vi "SCA state Transition Timeout Check.vi"(6 "Start Time":u32, 9 "Timeout limit":u32, 10 "Current State In":T1, 11 "Modified Array of states in":T1[](array[typedef])) -> (0 "Status Message":string, 1 "millisecond timer value out":u32, 2 "Next State":T1, 3 "Modified Array of states out":T1[](array[typedef]))   [LabVIEW 2016]
doc: "Tranision Timeout Check takes the current state, modified array of states, timeout limit, and start time to: \n\n(1) determine if process has timed out\n(2) what state to progress to next, and \n(3) what the current status message should be."
uses:
  controls/SCA states.ctl
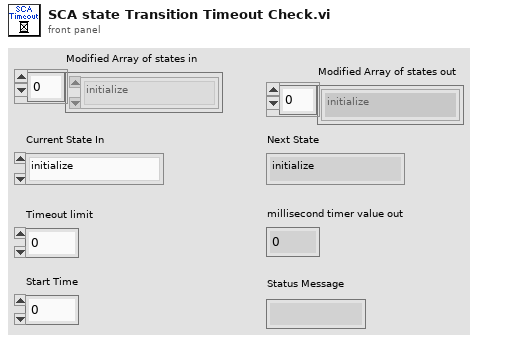
[diagram p1: front panel]
types:
  T1 = typedef "SCA states.ctl" = enum16{"initialize", "wait", "change sample start", "change sample", "check position", "rotate wheel", "sample change complete", "sample rod up", "sample rod down", "retract rod in", "retract rod out", "insert rod in", "insert rod out", "wheel GV open", "wheel GV close", "vent source", "pump source", "shutdown"}
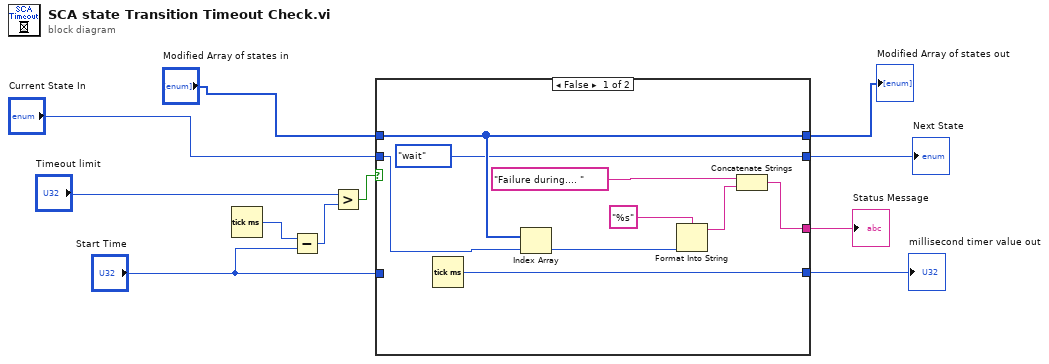
[diagram p0: block diagram]
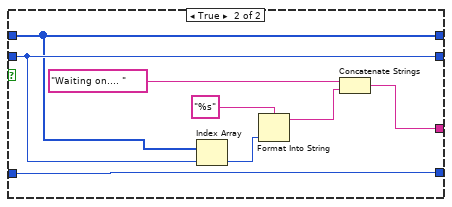
[diagram p2: hidden frame]
diagram:
  n1 = Tick Count (ms)() -> (millisecond timer value=w6:u32)
  n2 = Subtract(x=w6, y="Start Time") -> (x-y=w7:u32)
  n3 = Greater?(x="Timeout limit", y=w7) -> (0:w8:bool)
  n4 = case shown="False" w8 {
    tunnel: "Current State In" -> [w18 w27]
    tunnel: [SCA_states."wait" ("SCA state") w27] -> w4
    tunnel: "Modified Array of states in" -> [w16 w24]
    tunnel: [w16 w24] -> w1
    tunnel: "Start Time" -> [_ w28]
    tunnel: [w20 w28] -> w10
    tunnel: [w17 w25] -> w5
    frame False {
      n5 = Tick Count (ms)() -> (millisecond timer value=w20:u32)
      n6 = Index Array(array=w16, index=w18) -> (element=w13:T1)
      n7 = Format Into String(format string="%s", w13) -> (resulting string=w12:string)  [unwired: 2 in, 1 out]
      n8 = Concatenate Strings("Failure during.... ", w12) -> (w17:string)
    }
    frame True {
      n9 = Index Array(array=w24, index=w27) -> (element=w22:T1)
      n10 = Format Into String(format string="%s", w22) -> (resulting string=w21:string)  [unwired: 2 in, 1 out]
      n11 = Concatenate Strings("Waiting on.... ", w21) -> (w25:string)
    }
  }
  "millisecond timer value out" <- w10
  "Status Message" <- w5
  "Next State" <- w4
  "Modified Array of states out" <- w1
